vi "Stimulus.Open.vi"(8 "error in (no error)":errorcluster, 11 "State Variables":T1={"Events.State"=refnum, "Events.Test Result"=refnum, "Events.Progress"=refnum, "INI.Settings"={"Build Location"=path "C:/Simple Sequence Editor/SequenceRepo", "LoggingLocation"=path "", "Sequence.AbortChannel"="", "Sequence.IterationInfoChannel"="", "Sequence.DurationChannel"="", "Sequence.StepInfoChannel"="", "Sequence.SkipChannel"="", "PlotChannels"=[], "Sequence.InitializeScript"=path "C:/Simple Sequence Editor/SequenceRepo", "Sequence.CleanupScript"=path "", "Log.DefaultRate"=0.0}, "NIVS.AlarmManager"=refnum, "NIVS.BaseLogPath"=path "", "NIVS.DataLogManagerRef"=refnum, "NIVS.DataLogSpecRef"=refnum, "NIVS.Deployed"=FALSE, "NIVS.Events"={"SequenceEvent"=refnum, "SystemChangeEvent"=refnum, "WorkspaceEvent"=refnum}, "NIVS.GatewayIPAddress"="", "NIVS.DataLogGUID"="", "NIVS.ProfileCallback"=refnum, "NIVS.ProfileRef"=refnum, "NIVS.SequenceState"=enum."Idle", "NIVS.SystemDefinitionFile"=path "", "NIVS.SystemStateRefs"={"CustDatRef"=refnum, "EvtRef"=refnum, "Target State User Event"=refnum}, "NIVS.WorkspaceManager"=refnum, "NIVS.EventLogGUID"="", "NIVS.EventLogManagerRef"=refnum, "NIVS.EventLogSpecRef"=refnum, "NIVS.BaseToolPath"=path "", "Restart.Path"=path "", "Sequence.#ofColumns"=0, "Sequence.Iterations"=0, "Sequence.Channels"=[], "Sequence.ValidConfig?"=FALSE, "Station.ID"="", "UDP.Queue"=refnum, "UI.Abort"=refnum, "UI.Alarms"=refnum, "UI.Apply"=refnum, "UI.Back"=refnum, "UI.BaseFileName"=refnum, "UI.CurrentIteration"=refnum, "UI.CurrentStep"=refnum, "UI.CyclicFrequency"=refnum, "UI.Description"=refnum, "UI.DelayTime"=refnum, "UI.DisableAlarms"=refnum, "UI.Duration"=refnum, "UI.EnableLogging"=refnum, "UI.EnableState"=refnum, "UI.High"=refnum, "UI.LogChannels"=refnum, "UI.Low"=refnum, "UI.MonitoredVariable"=refnum, "UI.Next"=refnum, "UI.NumberOfCycles"=refnum, "UI.OperatorName"=refnum, "UI.Pause"=refnum, "UI.Profile"=refnum, "UI.Revert"=refnum, "UI.Skip"=refnum, "UI.Start"=refnum, "UI.StartIteration"=refnum, "UI.StartStep"=refnum, "UI.TabControl"=refnum, "UI.TotalIterations"=refnum, "UI.WaveformDefinition"=refnum, "UI.WaveformPreview"=refnum, "UI.WorkOrderNumber"=refnum, "UI.Chart"=refnum, "UI.Status"=refnum, "UI.DataView"=refnum, "UI.Table"=refnum, "UI.Multihead"=refnum, "UI.ToolTab"=refnum, "UI.Result"=refnum, "UI.Log Path"=refnum, "UI.ReportPath"=refnum, "UI.RestartPath"=refnum, "UI.AlarmLog"=refnum}) -> (0 "error out":errorcluster, 3 "State Variables":T1={"Events.State"=refnum, "Events.Test Result"=refnum, "Events.Progress"=refnum, "INI.Settings"={"Build Location"=path "C:/Simple Sequence Editor/SequenceRepo", "LoggingLocation"=path "", "Sequence.AbortChannel"="", "Sequence.IterationInfoChannel"="", "Sequence.DurationChannel"="", "Sequence.StepInfoChannel"="", "Sequence.SkipChannel"="", "PlotChannels"=[], "Sequence.InitializeScript"=path "C:/Simple Sequence Editor/SequenceRepo", "Sequence.CleanupScript"=path "", "Log.DefaultRate"=0.0}, "NIVS.AlarmManager"=refnum, "NIVS.BaseLogPath"=path "", "NIVS.DataLogManagerRef"=refnum, "NIVS.DataLogSpecRef"=refnum, "NIVS.Deployed"=FALSE, "NIVS.Events"={"SequenceEvent"=refnum, "SystemChangeEvent"=refnum, "WorkspaceEvent"=refnum}, "NIVS.GatewayIPAddress"="", "NIVS.DataLogGUID"="", "NIVS.ProfileCallback"=refnum, "NIVS.ProfileRef"=refnum, "NIVS.SequenceState"=enum."Idle", "NIVS.SystemDefinitionFile"=path "", "NIVS.SystemStateRefs"={"CustDatRef"=refnum, "EvtRef"=refnum, "Target State User Event"=refnum}, "NIVS.WorkspaceManager"=refnum, "NIVS.EventLogGUID"="", "NIVS.EventLogManagerRef"=refnum, "NIVS.EventLogSpecRef"=refnum, "NIVS.BaseToolPath"=path "", "Restart.Path"=path "", "Sequence.#ofColumns"=0, "Sequence.Iterations"=0, "Sequence.Channels"=[], "Sequence.ValidConfig?"=FALSE, "Station.ID"="", "UDP.Queue"=refnum, "UI.Abort"=refnum, "UI.Alarms"=refnum, "UI.Apply"=refnum, "UI.Back"=refnum, "UI.BaseFileName"=refnum, "UI.CurrentIteration"=refnum, "UI.CurrentStep"=refnum, "UI.CyclicFrequency"=refnum, "UI.Description"=refnum, "UI.DelayTime"=refnum, "UI.DisableAlarms"=refnum, "UI.Duration"=refnum, "UI.EnableLogging"=refnum, "UI.EnableState"=refnum, "UI.High"=refnum, "UI.LogChannels"=refnum, "UI.Low"=refnum, "UI.MonitoredVariable"=refnum, "UI.Next"=refnum, "UI.NumberOfCycles"=refnum, "UI.OperatorName"=refnum, "UI.Pause"=refnum, "UI.Profile"=refnum, "UI.Revert"=refnum, "UI.Skip"=refnum, "UI.Start"=refnum, "UI.StartIteration"=refnum, "UI.StartStep"=refnum, "UI.TabControl"=refnum, "UI.TotalIterations"=refnum, "UI.WaveformDefinition"=refnum, "UI.WaveformPreview"=refnum, "UI.WorkOrderNumber"=refnum, "UI.Chart"=refnum, "UI.Status"=refnum, "UI.DataView"=refnum, "UI.Table"=refnum, "UI.Multihead"=refnum, "UI.ToolTab"=refnum, "UI.Result"=refnum, "UI.Log Path"=refnum, "UI.ReportPath"=refnum, "UI.RestartPath"=refnum, "UI.AlarmLog"=refnum})   [LabVIEW 2015, in "Single Station Execution.lvlib"]
uses:
  Single Station Execution.lvlib
  Types/Main.StateVariables.ctl
  Types/INI.Settings.ctl
  <vilib>/NI Veristand/Execution/AlarmManager/AlarmManagerAPI.ctl
  NationalInstruments.VeriStand.ClientAPI
  <vilib>/NI Veristand/Execution/DataLogging/IDataLogging Ref.ctl
  <vilib>/NI Veristand/Execution/DataLogging/DataLoggingSpecification Ref.ctl
  Types/Execute.UserEventRefs.ctl
  <vilib>/NI Veristand/Execution/Workspace/SystemStateRegEventRef.ctl
  <vilib>/NI Veristand/Execution/Workspace/Target State Info.ctl
  <vilib>/NI Veristand/Execution/Workspace/Target State.ctl
  NationalInstruments.VeriStand.RealTimeSequenceDefinitionApi
  Types/Execution.SequenceState.ctl
  <vilib>/NI Veristand/Execution/Workspace/SystemStateEventRef.ctl
  <vilib>/NI Veristand/Execution/Workspace/WorkspaceAPI.ctl
  Types/UDPEngine.QueueCluster.ctl
  Types/UDPEngine.State.ctl
  <vilib>/NI Veristand/Execution/DataLogging/TDMS Property.ctl
  NationalInstruments.VeriStand.DataTypes
  <vilib>/NI Veristand/Execution/DataLogging/File Conflict Operation.ctl
  <vilib>/NI Veristand/Execution/DataLogging/Slope.ctl
  Main.Constants.vi
  <vilib>/NI Veristand/Execution/DataLogging/New Data Logging Specification (TDMS).vi
  <vilib>/NI Veristand/Execution/DataLogging/Set Data Logging Rate (Custom Rate).vi
  <vilib>/NI Veristand/Execution/DataLogging/Set Data Logging Rate (Target Rate).vi
  <vilib>/NI Veristand/Execution/DataLogging/Set Start Trigger (Start Immediately).vi
  <vilib>/NI Veristand/Execution/DataLogging/Set Start Trigger (Digital Edge).vi
  <vilib>/NI Veristand/Execution/DataLogging/Set Stop Trigger (Duration).vi
  <vilib>/NI Veristand/Execution/DataLogging/NI_VS Data Logging API.lvlib
  <vilib>/NI Veristand/Execution/Workspace/NI_VS Workspace ExecutionAPI.lvlib
  <vilib>/NI Veristand/Execution/AlarmManager/NI_VS AlarmManager ExecutionAPI.lvlib
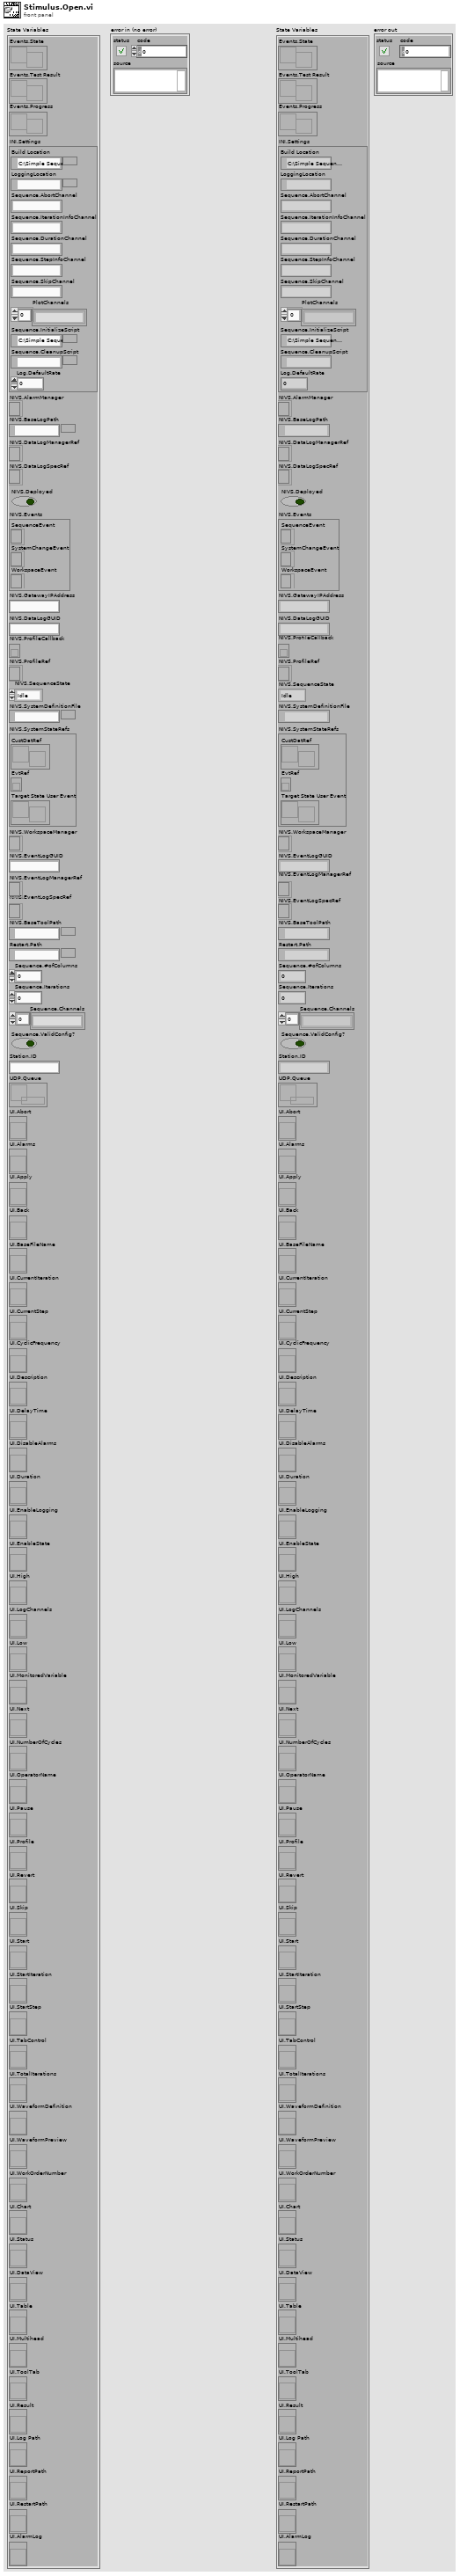
[diagram p1: front panel]
types:
  T1 = typedef "Single Station Execution.lvlib/Main.StateVariables.ctl" = cluster{"Events.State":refnum<user-event>, "Events.Test Result":refnum<user-event>, "Events.Progress":refnum<user-event>, "INI.Settings":T2, "NIVS.AlarmManager":T3, "NIVS.BaseLogPath":path, "NIVS.DataLogManagerRef":T4, "NIVS.DataLogSpecRef":T5, "NIVS.Deployed":bool, "NIVS.Events":T6, "NIVS.GatewayIPAddress":string, "NIVS.DataLogGUID":string, "NIVS.ProfileCallback":refnum<k27>, "NIVS.ProfileRef":refnum<k24>, "NIVS.SequenceState":T8, "NIVS.SystemDefinitionFile":path, "NIVS.SystemStateRefs":T9, "NIVS.WorkspaceManager":T10, "NIVS.EventLogGUID":string, "NIVS.EventLogManagerRef":T4, "NIVS.EventLogSpecRef":T5, "NIVS.BaseToolPath":path, "Restart.Path":path, "Sequence.#ofColumns":i32, "Sequence.Iterations":u32, "Sequence.Channels":string[], "Sequence.ValidConfig?":bool, "Station.ID":string, "UDP.Queue":refnum<queue>, "UI.Abort":refnum<vi>, "UI.Alarms":refnum<vi>, "UI.Apply":refnum<vi>, "UI.Back":refnum<vi>, "UI.BaseFileName":refnum<vi>, "UI.CurrentIteration":refnum<vi>, "UI.CurrentStep":refnum<vi>, "UI.CyclicFrequency":refnum<vi>, "UI.Description":refnum<vi>, "UI.DelayTime":refnum<vi>, "UI.DisableAlarms":refnum<vi>, "UI.Duration":refnum<vi>, "UI.EnableLogging":refnum<vi>, "UI.EnableState":refnum<vi>, "UI.High":refnum<vi>, "UI.LogChannels":refnum<vi>, "UI.Low":refnum<vi>, "UI.MonitoredVariable":refnum<vi>, "UI.Next":refnum<vi>, "UI.NumberOfCycles":refnum<vi>, "UI.OperatorName":refnum<vi>, "UI.Pause":refnum<vi>, "UI.Profile":refnum<vi>, "UI.Revert":refnum<vi>, "UI.Skip":refnum<vi>, "UI.Start":refnum<vi>, "UI.StartIteration":refnum<vi>, "UI.StartStep":refnum<vi>, "UI.TabControl":refnum<vi>, "UI.TotalIterations":refnum<vi>, "UI.WaveformDefinition":refnum<vi>, "UI.WaveformPreview":refnum<vi>, "UI.WorkOrderNumber":refnum<vi>, "UI.Chart":refnum<vi>, "UI.Status":refnum<vi>, "UI.DataView":refnum<vi>, "UI.Table":refnum<vi>, "UI.Multihead":refnum<vi>, "UI.ToolTab":refnum<vi>, "UI.Result":refnum<vi>, "UI.Log Path":refnum<vi>, "UI.ReportPath":refnum<vi>, "UI.RestartPath":refnum<vi>, "UI.AlarmLog":refnum<vi>}
  T2 = typedef "Single Station Execution.lvlib/INI.Settings.ctl" = cluster{"Build Location":path, "LoggingLocation":path, "Sequence.AbortChannel":string, "Sequence.IterationInfoChannel":string, "Sequence.DurationChannel":string, "Sequence.StepInfoChannel":string, "Sequence.SkipChannel":string, "PlotChannels":string[], "Sequence.InitializeScript":path, "Sequence.CleanupScript":path, "Log.DefaultRate":dbl}
  T3 = typedef "NI_VS AlarmManager ExecutionAPI.lvlib/AlarmManagerAPI.ctl" = refnum<k24>
  T4 = typedef "NI_VS Data Logging API.lvlib/IDataLogging Ref.ctl" = refnum<k24>
  T5 = typedef "NI_VS Data Logging API.lvlib/DataLoggingSpecification Ref.ctl" = refnum<k24>
  T6 = typedef "Single Station Execution.lvlib/Execute.UserEventRefs.ctl" = cluster{"SequenceEvent":refnum<event-registration>, "SystemChangeEvent":T7, "WorkspaceEvent":refnum<event-registration>}
  T7 = typedef "NI_VS Workspace ExecutionAPI.lvlib/SystemStateRegEventRef.ctl" = refnum<event-registration>
  T8 = typedef "Single Station Execution.lvlib/Execution.SequenceState.ctl" = enum16{"Idle", "Initializing", "Running", "Paused", "Finalizing", "Complete"}
  T9 = typedef "NI_VS Workspace ExecutionAPI.lvlib/SystemStateEventRef.ctl" = cluster{"CustDatRef":refnum<user-event>, "EvtRef":refnum<k27>, "Target State User Event":refnum<user-event>}
  T10 = typedef "NI_VS Workspace ExecutionAPI.lvlib/WorkspaceAPI.ctl" = refnum<k24>
  T11 = typedef "Single Station Execution.lvlib/Restart.Settings.ctl" = cluster{"LogFile":path, "Log Settings":T12[], "StimulusProfile":path, "StopIteration":u32, "StopStep":u32, "Log Channels":T16, "Base File Name":string, "Enable Logging":bool, "Profile":string, "StopDuration":dbl, "Waveform Definition":path, "Number of Cycles":dbl, "Cyclic Frequency":dbl, "Work Order Number":string, "Operator Name":string, "Description":string, "Station.ID":string, "Sequence.Channels":string[], "Alarms":T17[]}
  T12 = typedef "NI_VS Data Logging API.lvlib/TDMS Channel Group.ctl" = cluster{"Group Name":string, "Group Description":string, "Group Properties":T13[], "Channels":T14[], "Time Channel Options":T15, "Time Channel Name":string}
  T13 = typedef "NI_VS Data Logging API.lvlib/TDMS Property.ctl" = cluster{"Name":string, "Value":variant}
  T14 = typedef "NI_VS Data Logging API.lvlib/TDMS Channel.ctl" = cluster{"Channel Name":string, "Channel Path":string, "Channel Description":string, "Channel Properties":T13[]}
  T15 = typedef "NI_VS Data Logging API.lvlib/Time Channel Options.ctl" = enum16{"No Time Channel", "Absolute Time", "System Time", "System Time - Microseconds", "Absolute Time as Double"}
  T16 = typedef "Single Station Execution.lvlib/Log.SelectedChannels.ctl" = enum16{"Channels (No System Channel)", "Aliases", "All"}
  T17 = typedef "Single Station Execution.lvlib/Config.AlarmSettings.ctl" = cluster{"Watch Channel":string, "High Limit":dbl, "Low Limit":dbl, "Delay":dbl, "State":enum16{"Disabled", "Enabled", "Tripped", "Delayed Trip", "Indicate"}, "Alarm Name":string}
  T18 = typedef "NI_VS Data Logging API.lvlib/File Conflict Operation.ctl" = enum16{"Create Unique", "Append to Existing", "Overwrite"}
  T19 = typedef "NI_VS Data Logging API.lvlib/Slope.ctl" = enum16{"Rising", "Falling"}
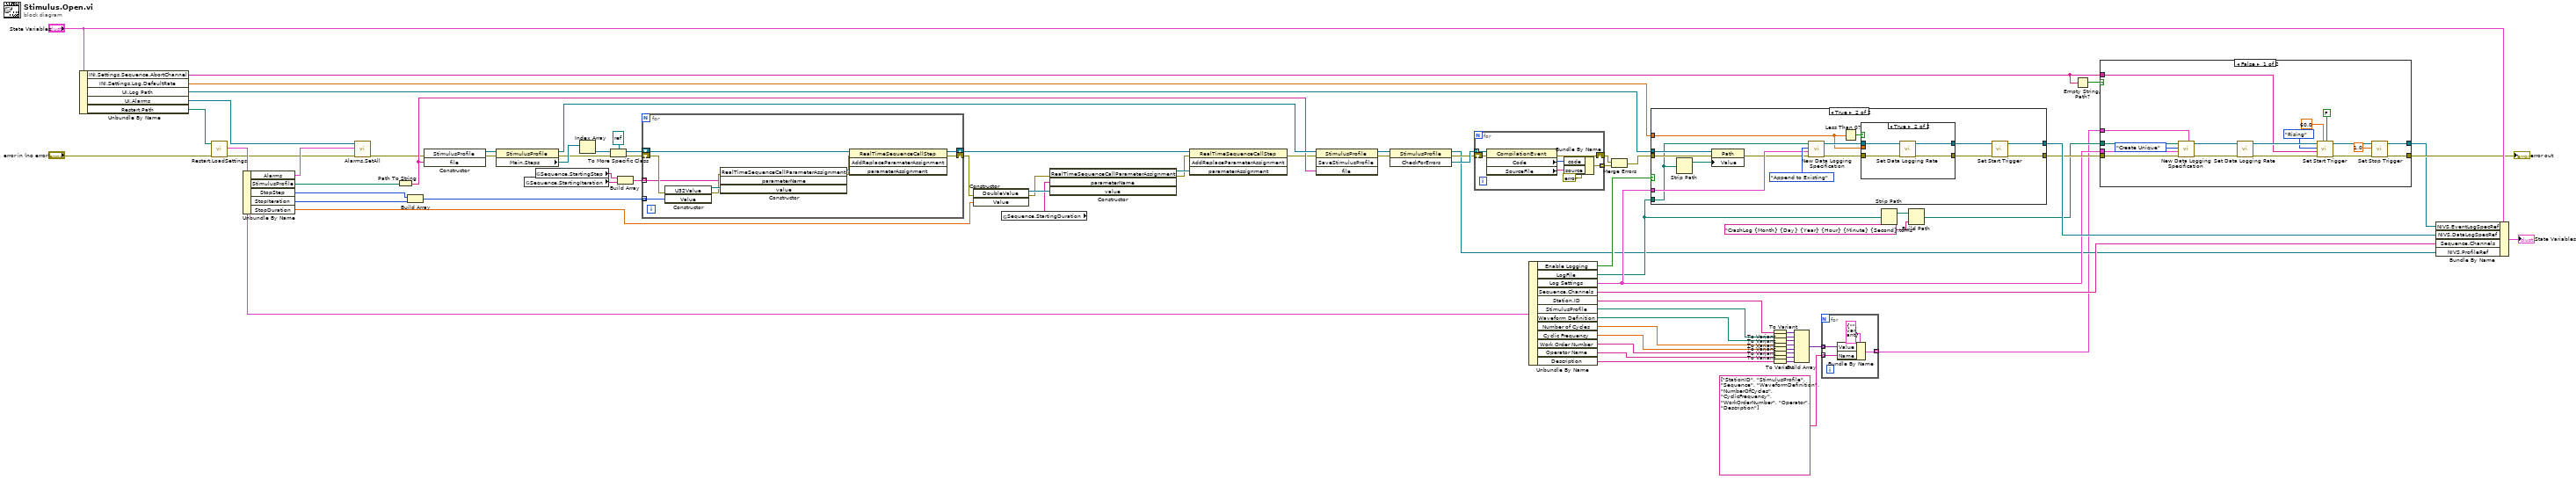
[diagram p0: block diagram]
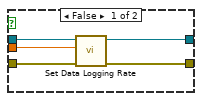
[diagram p4: hidden frame]
diagram:
  n1 = Unbundle By Name("State Variables") -> ("INI.Settings.Sequence.AbortChannel"=w24:string, "INI.Settings.Log.DefaultRate"=w36:dbl, "UI.Log Path"=w37:refnum<vi>, "UI.Alarms"=w4:refnum<vi>, "Restart.Path"=w62:path)
  n2 = call "Restart.LoadSettings.vi"("error in"="error in (no error)", "path (use dialog)"=w62) -> ("error out"=w2:errorcluster, "Restart Settings"=w49:T11)  [unwired: 7 in, 1 out]
  n3 = Unbundle By Name(w49) -> ("Alarms"=w3:T17[], "StimulusProfile"=w59:path, "StopStep"=w60:u32, "StopIteration"=w61:u32, "StopDuration"=w40:dbl)
  n4 = call "Alarms.SetAll.vi"("error in (no error)"=w2, "Alarms"=w3, "ListBox in"=w4) -> ("error out"=w1:errorcluster)  [unwired: 8 in]
  n5 = Path To String(path=w59) -> (string=w50:string)
  n6 = Build Array(w60, w61) -> (w52:u32[])
  n7 = constructor class="StimulusProfile"(error in=w1, "file"=w50) -> (reference out=w75:refnum<k24>, error out=w74:errorcluster)  [unwired: 2 in, 2 out]
  n8 = property class="StimulusProfile"(reference=w75, error in=w74) -> (reference out=w65:refnum<k24>, error out=w55:errorcluster, "Main.Steps"=w58:refnum<k24>[])
  n9 = global read "Main.Constants.vi" "Sequence.StartingIteration"() -> (w66:string)
  n10 = global read "Main.Constants.vi" "Sequence.StartingStep"() -> (w67:string)
  n11 = Index Array(array=w58) -> (element=w57:refnum<k24>)  [unwired: 1 in]
  n12 = To More Specific Class(target class=refnum<k24> refnum ("new reference"), reference=w57, error in=w55) -> (specific class reference=w54:refnum<k24>, error out=w51:errorcluster)
  n13 = Build Array(w67, w66) -> (w53:string[])
  n14 = for {
    tunnel: w53 -> [w80] mode=indexing
    tunnel: w52 -> [w78] mode=indexing
    shift-right: [w85] -> w41
    shift-left: w54 -> [w86]
    shift-right: [w87] -> w42
    shift-left: w51 -> [w81]
    n15 = constructor class="U32Value"(error in=w81, "Value"=w78) -> (reference out=w83:refnum<k24>, error out=w82:errorcluster)  [unwired: 2 in, 2 out]
    n16 = constructor class="RealTimeSequenceCallParameterAs"(error in=w82, "parameterName"=w80, "value"=w83) -> (reference out=w84:refnum<k24>, error out=w79:errorcluster)  [unwired: 2 in, 3 out]
    n17 = invoke class="RealTimeSequenceCallStep" method="AddReplaceParameterAssignment"(reference=w86, error in=w79, "parameterAssignment"=w84) -> (reference out=w85:refnum<k24>, error out=w87:errorcluster)  [unwired: 1 in, 2 out]
  }
  n18 = constructor class="DoubleValue"(error in=w42, "Value"=w40) -> (reference out=w46:refnum<k24>, error out=w45:errorcluster)  [unwired: 2 in, 2 out]
  n19 = global read "Main.Constants.vi" "Sequence.StartingDuration"() -> (w39:string)
  n20 = constructor class="RealTimeSequenceCallParameterAs"(error in=w45, "parameterName"=w39, "value"=w46) -> (reference out=w47:refnum<k24>, error out=w44:errorcluster)  [unwired: 2 in, 3 out]
  n21 = invoke class="RealTimeSequenceCallStep" method="AddReplaceParameterAssignment"(reference=w41, error in=w44, "parameterAssignment"=w47) -> (error out=w43:errorcluster)  [unwired: 1 in, 3 out]
  n22 = invoke class="StimulusProfile" method="SaveStimulusProfile"(reference=w65, error in=w43, "file"=w50) -> (reference out=w73:refnum<k24>, error out=w72:errorcluster)  [unwired: 1 in, 2 out]
  n23 = invoke class="StimulusProfile" method="CheckForErrors"(reference=w73, error in=w72) -> (reference out=w25:refnum<k24>, error out=w70:errorcluster, "CheckForErrors"=w71:refnum<k24>[])  [unwired: 1 in]
  n24 = for {
    tunnel: w71 -> [w94] mode=indexing
    tunnel: [w89] -> w68 mode=indexing
    shift-right: [w88] -> w69
    shift-left: w70 -> [w93]
    n25 = property class="CompilationEvent"(reference=w94, error in=w93) -> (error out=w88:errorcluster, "Code"=w91:i32, "SourceFile"=w90:string)  [unwired: 1 out]
    n26 = Bundle By Name(cluster=errorcluster {"status"=TRUE, "code"=0, "source"=""} ("error out"), "code"=w91, "source"=w90) -> (w89:errorcluster)
  }
  n27 = Unbundle By Name(w49) -> ("Enable Logging"=w26:bool, "LogFile"=w29:path, "Log Settings"=w32:T12[], "Sequence.Channels"=w38:string[], "Station.ID"=w6:string, "StimulusProfile"=w7:path, "Waveform Definition"=w8:path, "Number of Cycles"=w9:dbl, "Cyclic Frequency"=w10:dbl, "Work Order Number"=w11:string, "Operator Name"=w12:string, "Description"=w13:string)
  n28 = Merge Errors(w69, w68) -> (w48:errorcluster)
  n29 = case shown="True" w26 {
    tunnel: w48 -> [w95 w102]
    tunnel: [w95 w105] -> w34
    tunnel: [_ w104] -> w64
    tunnel: w29 -> [_ w96]
    tunnel: w32 -> [_ w103]
    tunnel: w37 -> [_ w100]
    tunnel: w36 -> [_ w98]
    frame False {
    }
    frame True {
      n30 = Strip Path(path=w96) -> (stripped path=w97:path)  [unwired: 1 out]
      n31 = property class="Path"(reference=w100, error in=w102, "Value"=w97) -> (error out=w101:errorcluster)  [unwired: 1 out]
      n32 = call-poly <vilib>:"New Data Logging Specification.vi"("error in (no error)"=w101, "Channel Groups"=w103, "File Conflict Operation"=File_Conflict_Operation."Append to Existing", "Base Log File Path"=w96) -> ("error out"=w107:errorcluster, "Data Logging Specification Ref out"=w110:T5)  [unwired: 6 in]
      n33 = Less Than 0?(x=w98) -> (x < 0?=w99:bool)
      n34 = case shown="True" w99 {
        tunnel: w110 -> [w115 w119]
        tunnel: [w112 w118] -> w109
        tunnel: [w113 w117] -> w108
        tunnel: w107 -> [w114 w116]
        tunnel: w98 -> [w111 _]
        frame False {
          n35 = call-poly <vilib>:"Set Data Logging Rate.vi"("error in (no error)"=w114, "Custom Rate (Hz)"=w111, "Data Logging Specification Ref in"=w115) -> ("error out"=w113:errorcluster, "Data Logging Specification Ref out"=w112:T5)  [unwired: 7 in]
        }
        frame True {
          n36 = call-poly <vilib>:"Set Data Logging Rate.vi"("error in (no error)"=w116, "Data Logging Specification Ref in"=w119) -> ("error out"=w117:errorcluster, "Data Logging Specification Ref out"=w118:T5)  [unwired: 8 in]
        }
      }
      n37 = call-poly <vilib>:"Set Start Trigger.vi"("error in (no error)"=w108, "Data Logging Specification Ref in"=w109) -> ("error out"=w105:errorcluster, "Data Logging Specification Ref out"=w104:T5)  [unwired: 8 in]
    }
  }
  n38 = To Variant(anything=w6) -> (Variant=w23:variant)
  n39 = To Variant(anything=w7) -> (Variant=w22:variant)
  n40 = To Variant(anything=w8) -> (Variant=w21:variant)
  n41 = To Variant(anything=w9) -> (Variant=w20:variant)
  n42 = To Variant(anything=w10) -> (Variant=w19:variant)
  n43 = To Variant(anything=w11) -> (Variant=w18:variant)
  n44 = To Variant(anything=w12) -> (Variant=w17:variant)
  n45 = To Variant(anything=w13) -> (Variant=w16:variant)
  n46 = Build Array(w23, w22, w21, w20, w19, w18, w17, w16) -> (w15:variant[])
  n47 = for {
    tunnel: w15 -> [w123] mode=indexing
    tunnel: string[] ["StationID", "StimulusProfile", "Sequence", "WaveformDefinition", "NumberOfCycles", "CyclicFrequency", "WorkOrderNumber", "Operator", "Description"] -> [w121] mode=indexing
    tunnel: [w120] -> w5 mode=indexing
    n48 = Bundle By Name(cluster=T13 {"Name"="", "Value"=variant} ("TDMS Property"), "Value"=w123, "Name"=w121) -> (w120:T13)
  }
  n49 = Strip Path(path=w29) -> (stripped path=w28:path)  [unwired: 1 out]
  n50 = Build Path(base path=w28, name or relative path="CrashLog {Month} {Day} {Year} {Hour} {Minute} {Second}.tdms") -> (appended path=w27:path)
  n51 = Empty String/Path?(string/path=w24) -> (empty?=w35:bool)
  n52 = case shown="False" w35 {
    tunnel: w34 -> [w129 w142]
    tunnel: [w126 w142] -> w33
    tunnel: w24 -> [w136 _]
    tunnel: [w125 _] -> w31
    tunnel: w32 -> [w128 _]
    tunnel: w27 -> [w127 _]
    tunnel: w5 -> [w124 _]
    frame False {
      n53 = call-poly <vilib>:"New Data Logging Specification.vi"("File Properties"=w124, "error in (no error)"=w129, "Channel Groups"=w128, "File Conflict Operation"=File_Conflict_Operation."Create Unique", "Base Log File Path"=w127) -> ("error out"=w140:errorcluster, "Data Logging Specification Ref out"=w137:T5)  [unwired: 5 in]
      n54 = call-poly <vilib>:"Set Data Logging Rate.vi"("error in (no error)"=w140, "Data Logging Specification Ref in"=w137) -> ("error out"=w139:errorcluster, "Data Logging Specification Ref out"=w138:T5)  [unwired: 8 in]
      n55 = call-poly <vilib>:"Set Start Trigger.vi"("Retriggerable (F)"=FALSE, "Pre-Trigger Duration (0 s)"=60.0, "error in (no error)"=w139, "Trigger Channel"=w136, "Slope"=Slope."Rising", "Data Logging Specification Ref in"=w138) -> ("error out"=w132:errorcluster, "Data Logging Specification Ref out"=w131:T5)  [unwired: 4 in]
      n56 = call-poly <vilib>:"Set Stop Trigger.vi"("error in (no error)"=w132, "Duration"=1.0, "Data Logging Specification Ref in"=w131) -> ("error out"=w126:errorcluster, "Data Logging Specification Ref out"=w125:T5)  [unwired: 7 in]
    }
    frame True {
    }
  }
  "error out" <- w33
  n57 = Bundle By Name(cluster="State Variables", "NIVS.EventLogSpecRef"=w31, "NIVS.DataLogSpecRef"=w64, "Sequence.Channels"=w38, "NIVS.ProfileRef"=w25) -> (→"State Variables":T1)
